vi "STM Read Msg.vi"(7 "Ignore Timeout Error":bool=TRUE, 8 "error in":errorcluster, 9 "Meta data":T1[](array[typedef]), 10 "timeout ms (25000)":i32=25000, 11 "connection ID":refnum<k5>) -> (0 "error out":errorcluster, 1 "Meta element":T1, 2 "data string":string, 3 "connection ID out":refnum<k5>, 4 "Data Size":i32, 5 "Timed Out?":bool)   [LabVIEW 2013]
doc: "This VI reads an incoming package of data from a host. This VI parses the package and extracts the data name and type as described in the meta data.\n\nFor the package to be parsed correctly, the meta data must be consistent in both the sender and the receiver. The data is packaged based on the existing meta data on the sender. \n\nUse the \"Read Meta\" and \"Write Meta\" VIs to ensure that both client and server have the same meta data.\n\nThe data is returned as a string. It is the responsibility of the user to cast it to the appropriate type."
uses:
  stm_MetaElement.ctl
  stm_MetaID.ctl
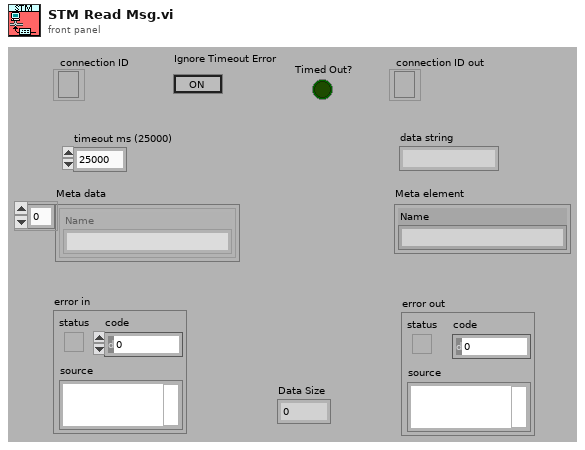
[diagram p1: front panel]
types:
  T1 = typedef "stm_MetaElement.ctl" = cluster{"Name":string}
  T2 = typedef "stm_MetaID.ctl" = u16
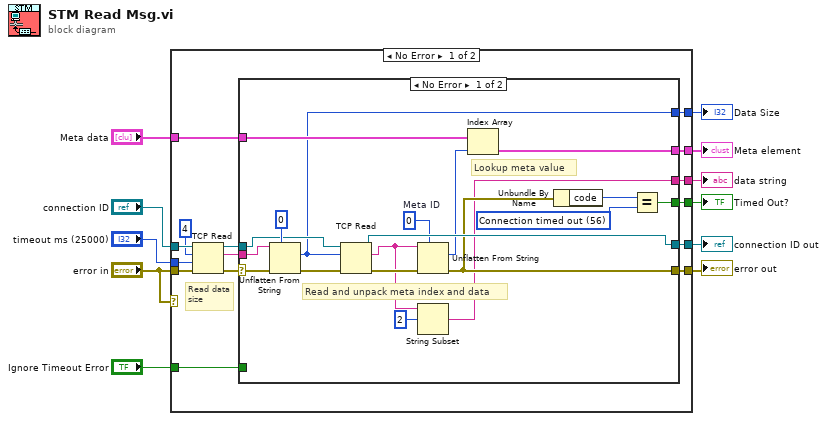
[diagram p0: block diagram]
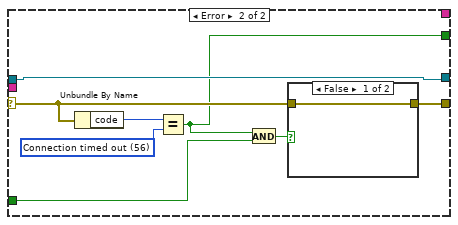
[diagram p2: hidden frame]
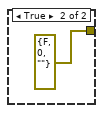
[diagram p3: hidden frame]
diagram:
  n1 = case shown="No Error" "error in" {
    tunnel: "error in" -> [w26 w56]
    tunnel: "connection ID" -> [w25 w57]
    tunnel: "Meta data" -> [w21 _]
    tunnel: "timeout ms (25000)" -> [w20 _]
    tunnel: [w18 w57] -> w8
    tunnel: [w17 w56] -> w7
    tunnel: "Ignore Timeout Error" -> [w16 _]
    tunnel: [w15 _] -> w5
    tunnel: [w14 _] -> w4
    tunnel: [w13 _] -> w3
    tunnel: [w12 _] -> w1
    frame No Error {
      # "Read data size"
      n2 = TCP Read(connection ID=w25, bytes to read=4, error in (no error)=w26, 9:w20) -> (connection ID out=w22:refnum<k5>, data out=w23:string, error out=w19:errorcluster)  [unwired: 1 out]
      n3 = case shown="No Error" w19 {
        selector: w19 -> [w36 w47]
        tunnel: w23 -> [w37 _]
        tunnel: w22 -> [w44 w53]
        tunnel: w21 -> [w43 _]
        tunnel: [w42 w53] -> w18
        tunnel: [w33 w48] -> w17
        tunnel: w16 -> [_ w50]
        tunnel: [w39 w46] -> w15
        tunnel: [w32 _] -> w14
        tunnel: [w27 _] -> w13
        tunnel: [w31 _] -> w12
        frame No Error {
          w30 = T2 0  # Meta ID
          w40 = 56 items=["No Error", "Argument Error", "Memory Full", "Out of Zone", "End of File", "File Already Open", "Generic File IO Error", "File Not Found", "File Permission Error", "Disk Full", "Duplicate Path", "Too Many Files Open", "Not Enabled", "Resource File Not Found", "Cannot Add Resource", "Resource Not Found", "Image Not Found", "Image Memory Error", "Pen Does Not Exist", "Config Bad Type", "Config Token Not Found", "Config Parse Error", "Config Memory Error", "Bad External Code Format", "Bad External Code Offset", "External Code Not Present", "Null Window", "Destroy Window Mixup", "Null Menu", "Print Aborted", "Bad Print Record", "Print Driver Error", "Windows Error During Print", "Memory Error During Print", "Print Dialog Error", "Generic Print Error", "Invalid Device Refnum", "Device Not Found", "Device Parameter Error", "Device Unit Error", "Can't Open Device", "Device Call Aborted", "Generic Error", "Cancelled By User", "Object ID Too Low", "Object ID Too High", "Object Not In Heap", "Unknown Heap", "Bad DefProc ID", "DefProc Not In Table", "Message Out Of Range", "Null Method", "Unknown Message", "Manager Call Not Supported", "Bad address", "Connection In progress", "Connection timed out", "Connection is already in progress", "Network attribute not supported", "Network error", "Address in use", "System out of memory", "Connection aborted", "Connection refused", "Connection is not connected", "Connection is already connected", "Connection closed", "Initialize error (interapplication manager)", "Bad occurrence", "Wait on unbound occurrence handler", "Occurrence queue overflow", "Bad path", "Semaphore not signaled", "Unrecognized type (interapplication manager)"] ("1st Error to Convert")
          # "Lookup meta value"
          # "Read and unpack meta index and data"
          n4 = Unflatten From String(type=0 ("bytes to read"), binary string=w37, error in (no error)=w36) -> (value=w31:i32, error out=w35:errorcluster)  [unwired: 1 in, 2 out]
          n5 = TCP Read(connection ID=w44, bytes to read=w31, error in (no error)=w35) -> (connection ID out=w42:refnum<k5>, data out=w28:string, error out=w34:errorcluster)  [unwired: 2 out]
          n6 = Unflatten From String(type=w30, binary string=w28, error in (no error)=w34) -> (value=w38:T2, error out=w33:errorcluster)  [unwired: 3 out]
          n7 = String Subset(string=w28, offset (0)=2) -> (substring=w27:string)  [unwired: 1 out]
          n8 = Index Array(array=w43, index=w38) -> (element=w32:T1)
          n9 = Unbundle By Name(w33) -> ("code"=w41:i32)
          n10 = Equal?(x=w41, y=w40) -> (x = y?=w39:bool)
        }
        frame Error {
          w51 = 56 items=["No Error", "Argument Error", "Memory Full", "Out of Zone", "End of File", "File Already Open", "Generic File IO Error", "File Not Found", "File Permission Error", "Disk Full", "Duplicate Path", "Too Many Files Open", "Not Enabled", "Resource File Not Found", "Cannot Add Resource", "Resource Not Found", "Image Not Found", "Image Memory Error", "Pen Does Not Exist", "Config Bad Type", "Config Token Not Found", "Config Parse Error", "Config Memory Error", "Bad External Code Format", "Bad External Code Offset", "External Code Not Present", "Null Window", "Destroy Window Mixup", "Null Menu", "Print Aborted", "Bad Print Record", "Print Driver Error", "Windows Error During Print", "Memory Error During Print", "Print Dialog Error", "Generic Print Error", "Invalid Device Refnum", "Device Not Found", "Device Parameter Error", "Device Unit Error", "Can't Open Device", "Device Call Aborted", "Generic Error", "Cancelled By User", "Object ID Too Low", "Object ID Too High", "Object Not In Heap", "Unknown Heap", "Bad DefProc ID", "DefProc Not In Table", "Message Out Of Range", "Null Method", "Unknown Message", "Manager Call Not Supported", "Bad address", "Connection In progress", "Connection timed out", "Connection is already in progress", "Network attribute not supported", "Network error", "Address in use", "System out of memory", "Connection aborted", "Connection refused", "Connection is not connected", "Connection is already connected", "Connection closed", "Initialize error (interapplication manager)", "Bad occurrence", "Wait on unbound occurrence handler", "Occurrence queue overflow", "Bad path", "Semaphore not signaled", "Unrecognized type (interapplication manager)"] ("1st Error to Convert")
          n11 = Unbundle By Name(w47) -> ("code"=w52:i32)
          n12 = Equal?(x=w52, y=w51) -> (x = y?=w46:bool)
          n13 = And(x=w46, y=w50) -> (x .and. y?=w49:bool)
          n14 = case shown="False" w49 {
            tunnel: [w54 errorcluster {"status"=FALSE, "code"=0, "source"=""} ("error out")] -> w48
            tunnel: w47 -> [w54 _]
            frame False {
            }
            frame True {
            }
          }
        }
      }
    }
    frame Error {
    }
  }
  "error out" <- w7
  "connection ID out" <- w8
  "Timed Out?" <- w5
  "data string" <- w3
  "Meta element" <- w4
  "Data Size" <- w1
